vi "Update Menu Theme List.vi"(8 "error in (no error)":errorcluster, 9 "Result":T1, 10 "Theme Name":string, 11 "Menu in":refnum<k9>) -> (0 "error out":errorcluster)   [LabVIEW 2021, in "Notebook.lvlib"]
uses:
  Notebook.lvlib
  Notebook Theme Edit Result.ctl
  Notebook Parameters List.ctl
panel:
  # "see the License on the block diagram (Ctrl+E or Window:Show Block Diagram)"
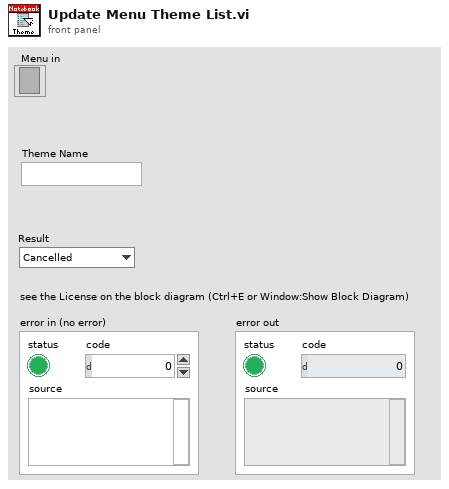
[diagram p1: front panel]
types:
  T1 = typedef "Notebook.lvlib/Notebook Theme Edit Result.ctl" = enum16{"Cancelled", "Modified Theme", "New Theme", "Remove Theme"}
  T2 = typedef "Notebook.lvlib/Notebook Parameters List.ctl" = enum16{"First Opening?", "Saved Notebook?", "Saved Notebook Path", "Beep on Error?", "Notebook Themes", "Current Theme Name"}
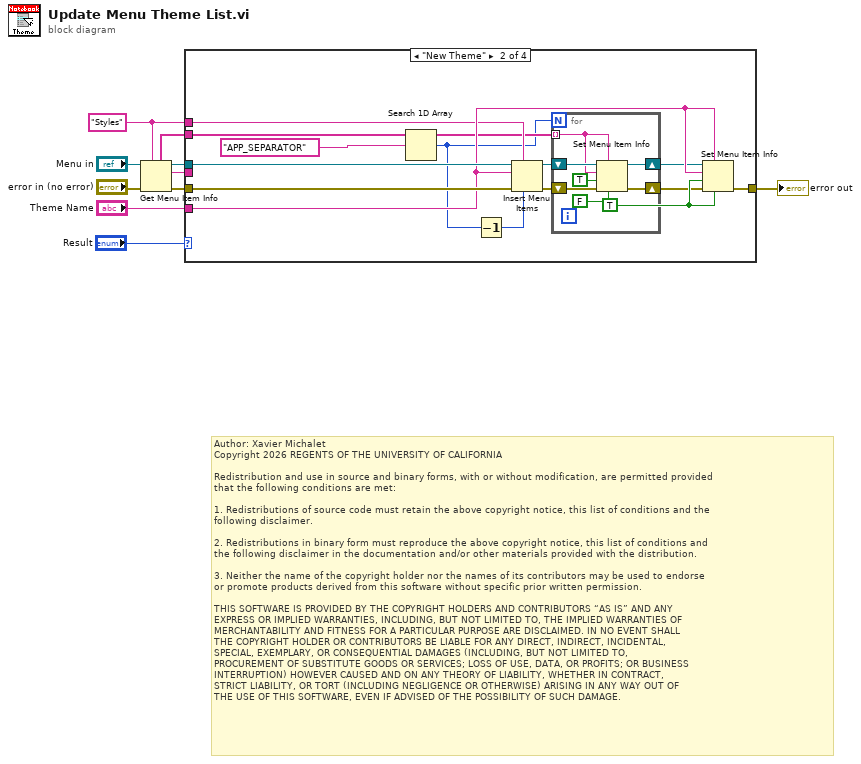
[diagram p0: block diagram]
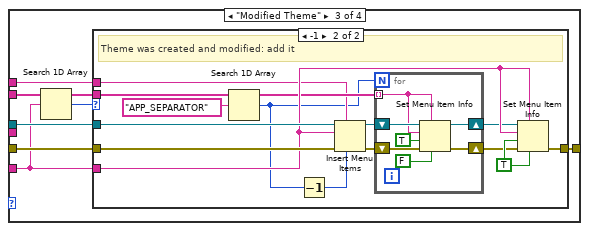
[diagram p3: hidden frame]
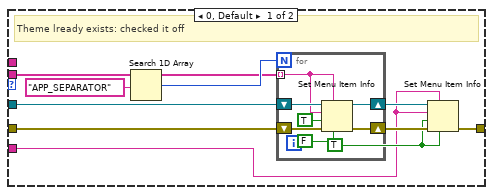
[diagram p4: hidden frame]
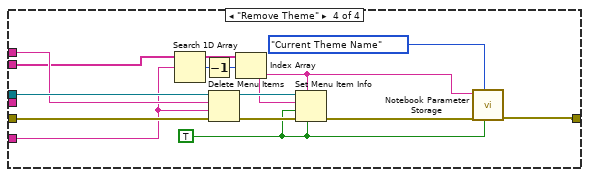
[diagram p5: hidden frame]
diagram:
  w4 = "Styles" ("item tag")
  # "Author: Xavier Michalet\nCopyright 2026 REGENTS OF THE UNIVERSITY OF CALIFORNIA\n\nRedistribution and use in source and binary forms, with or without modification, are permitted provided\nthat the following conditions are met:\n\n1. Redistributions of source code must retain the above copyright notice, this list of conditions and the\nfollowing disclaimer.\n\n2. Redistributions in binary form must reproduce the above copyright notice, this list of conditions and\nthe following disclaimer in the documentation and/or other materials provided with the distribution.\n\n3. Neither the name of the copyright holder nor the names of its contributors may be used to endorse \nor promote products derived from this software without specific prior written permission.\n\nTHIS SOFTWARE IS PROVIDED BY THE COPYRIGHT HOLDERS AND CONTRIBUTORS “AS IS” AND ANY \nEXPRESS OR IMPLIED WARRANTIES, INCLUDING, BUT NOT LIMITED TO, THE IMPLIED WARRANTIES OF\nMERCHANTABILITY AND FITNESS FOR A PARTICULAR PURPOSE ARE DISCLAIMED. IN NO EVENT SHALL\nTHE COPYRIGHT HOLDER OR CONTRIBUTORS BE LIABLE FOR ANY DIRECT, INDIRECT, INCIDENTAL, \nSPECIAL, EXEMPLARY, OR CONSEQUENTIAL DAMAGES (INCLUDING, BUT NOT LIMITED TO, \nPROCUREMENT OF SUBSTITUTE GOODS OR SERVICES; LOSS OF USE, DATA, OR PROFITS; OR BUSINESS\nINTERRUPTION) HOWEVER CAUSED AND ON ANY THEORY OF LIABILITY, WHETHER IN CONTRACT, \nSTRICT LIABILITY, OR TORT (INCLUDING NEGLIGENCE OR OTHERWISE) ARISING IN ANY WAY OUT OF\nTHE USE OF THIS SOFTWARE, EVEN IF ADVISED OF THE POSSIBILITY OF SUCH DAMAGE."
  n1 = Get Menu Item Info(7:w4, 8:"error in (no error)", 11:"Menu in") -> (0:w6:errorcluster, 2:w3:string, 3:w7:refnum<k9>, 5:w2:string[])  [unwired: 3 out]
  n2 = case shown="\"New Theme\"" "Result" {
    tunnel: "Theme Name" -> [_ w20 w36 w86]
    tunnel: w7 -> [_ w25 w39 w91]
    tunnel: w6 -> [w11 w22 w38 w90]
    tunnel: w4 -> [_ w18 w34 w89]
    tunnel: w3 -> [_ _ _ _]
    tunnel: w2 -> [_ w13 w35 w85]
    tunnel: [w11 w21 w37 w81] -> w1
    frame "Cancelled", Default {
    }
    frame "New Theme" {
      w19 = TRUE ("checked")
      n3 = Search 1D Array(1D array=w13, element="APP_SEPARATOR") -> (index of element=w12:i32)  [unwired: 1 in]
      n4 = Decrement(x=w12) -> (x-1=w23:i32)
      n5 = Insert Menu Items(4:w23, 5:w18, 6:w22, 8:w20, 9:w25) -> (0:w15:errorcluster, 3:w17:refnum<k9>)  [unwired: 1 in, 1 out]
      n6 = for {
        N: w12 -> [_]
        shift-right: [w31] -> w16
        shift-left: w17 -> [w32]
        shift-right: [w29] -> w14
        shift-left: w15 -> [w30]
        tunnel: w13 -> [w28] mode=indexing
        n7 = Set Menu Item Info(6:FALSE ("checked"), 7:w28, 8:w30, 9:TRUE ("enabled"), 10:w28, 11:w32) -> (0:w29:errorcluster, 3:w31:refnum<k9>)  [unwired: 1 in]
      }
      n8 = Set Menu Item Info(6:w19, 7:w20, 8:w14, 9:w19, 10:w20, 11:w16) -> (0:w21:errorcluster)  [unwired: 1 in, 1 out]
    }
    frame "Modified Theme" {
      n9 = Search 1D Array(1D array=w35, element=w36) -> (index of element=w33:i32)  [unwired: 1 in]
      n10 = case shown="-1" w33 {
        tunnel: w39 -> [w42 w70]
        tunnel: w38 -> [w43 w69]
        tunnel: [w40 w68] -> w37
        tunnel: w36 -> [w41 w67]
        tunnel: w35 -> [w44 w66]
        tunnel: w34 -> [_ w65]
        frame 0, Default {
          w46 = TRUE ("checked")
          # "Theme lready exists: checked it off"
          n11 = Search 1D Array(1D array=w44, element="APP_SEPARATOR") -> (index of element=w47:i32)  [unwired: 1 in]
          n12 = for {
            N: w47 -> [_]
            shift-right: [w55] -> w49
            shift-left: w42 -> [w56]
            shift-right: [w53] -> w48
            shift-left: w43 -> [w54]
            tunnel: w44 -> [w52] mode=indexing
            n13 = Set Menu Item Info(6:FALSE ("checked"), 7:w52, 8:w54, 9:TRUE ("enabled"), 10:w52, 11:w56) -> (0:w53:errorcluster, 3:w55:refnum<k9>)  [unwired: 1 in]
          }
          n14 = Set Menu Item Info(6:w46, 7:w41, 8:w48, 9:w46, 10:w41, 11:w49) -> (0:w40:errorcluster)  [unwired: 1 in, 1 out]
        }
        frame -1 {
          w62 = TRUE ("checked")
          # "Theme was created and modified: add it"
          n15 = Search 1D Array(1D array=w66, element="APP_SEPARATOR") -> (index of element=w57:i32)  [unwired: 1 in]
          n16 = Decrement(x=w57) -> (x-1=w63:i32)
          n17 = Insert Menu Items(4:w63, 5:w65, 6:w69, 8:w67, 9:w70) -> (0:w59:errorcluster, 3:w61:refnum<k9>)  [unwired: 1 in, 1 out]
          n18 = for {
            N: w57 -> [_]
            shift-right: [w76] -> w60
            shift-left: w61 -> [w77]
            shift-right: [w74] -> w58
            shift-left: w59 -> [w75]
            tunnel: w66 -> [w73] mode=indexing
            n19 = Set Menu Item Info(6:FALSE ("checked"), 7:w73, 8:w75, 9:TRUE ("enabled"), 10:w73, 11:w77) -> (0:w74:errorcluster, 3:w76:refnum<k9>)  [unwired: 1 in]
          }
          n20 = Set Menu Item Info(6:w62, 7:w67, 8:w58, 9:w62, 10:w67, 11:w60) -> (0:w68:errorcluster)  [unwired: 1 in, 1 out]
        }
      }
    }
    frame "Remove Theme" {
      w78 = TRUE ("enabled")
      n21 = Search 1D Array(1D array=w85, element=w86) -> (index of element=w84:i32)  [unwired: 1 in]
      n22 = Decrement(x=w84) -> (x-1=w83:i32)
      n23 = Delete Menu Items(6:w90, 7:w86, 8:w89, 9:w91) -> (0:w88:errorcluster, 3:w87:refnum<k9>)
      n24 = Index Array(array=w85, index=w83) -> (element=w79:string)
      n25 = Set Menu Item Info(6:w78, 7:w79, 8:w88, 9:w78, 10:w79, 11:w87) -> (0:w82:errorcluster)  [unwired: 1 in, 1 out]
      n26 = call "Notebook Parameter Storage.vi"("Get(F)/Set"=w78, "Notebook Parameter List"=Notebook_Parameters_List."Current Theme Name", "Error In"=w82, "Data in"=w79) -> ("Error Out"=w81:errorcluster)  [unwired: 6 in, 1 out]
    }
  }
  "error out" <- w1
